vi "Joint Saturation.vi"(10 "Joint Bounds [Deg/mm]":dbl[][](array[numeric])=[[-10.0, 35.0, 0.0, 0.0], [-35.0, -35.0, 0.0, 0.0], [0.5, 10.0, 0.0, 0.0], [-40.0, 40.0, 0.0, 0.0]], 11 "Ref Array [Deg/mm]":dbl[](array[numeric])=[0.0, 0.0, 0.0, 0.0]) -> (3 "Sat Ref Array [Deg/mm]":dbl[](array[numeric]))   [LabVIEW 2016]
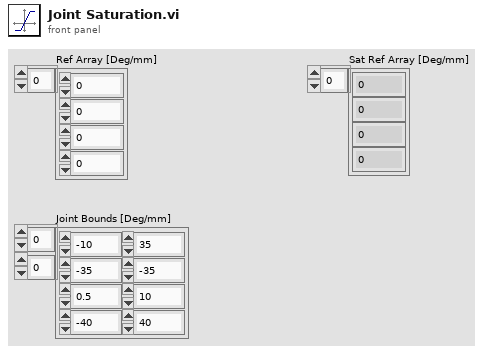
[diagram p1: front panel]
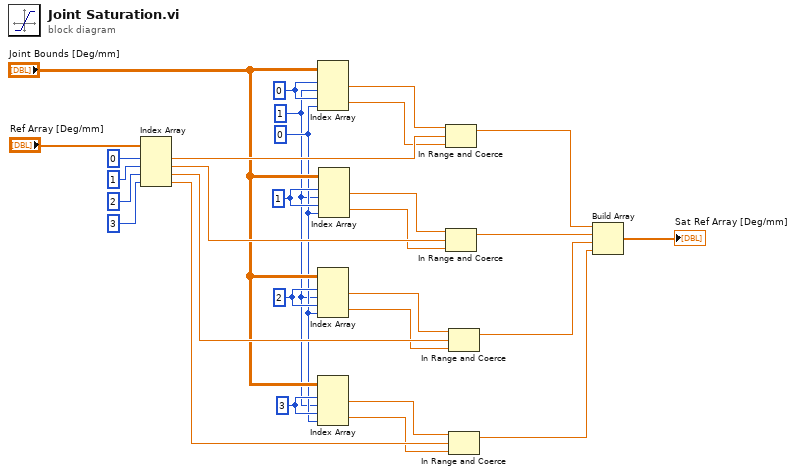
[diagram p0: block diagram]
diagram:
  w5 = 3 ("index (row)")
  w9 = 2
  w16 = 1 ("index (row)")
  w3 = 1 ("disabled index (col)")
  w4 = 0 ("index")
  w20 = 0 ("index")
  n1 = Index Array(array="Ref Array [Deg/mm]", index #1=0 ("index"), index #2=1 ("index"), index #3=2 ("index"), index #4=3 ("index")) -> (element #1=w24:dbl, element #2=w23:dbl, element #3=w22:dbl, element #4=w21:dbl)
  n2 = Index Array(array="Joint Bounds [Deg/mm]", index (row) #1=w20, index (col) #1=w3, index (row) #2=w20, index (col) #2=w4) -> (element #1=w19:dbl, element #2=w18:dbl)
  n3 = Index Array(array="Joint Bounds [Deg/mm]", index (row) #1=w9, index (col) #1=w3, index (row) #2=w9, index (col) #2=w4) -> (element #1=w8:dbl, element #2=w7:dbl)
  n4 = Index Array(array="Joint Bounds [Deg/mm]", index (row) #1=w5, index (col) #1=w3, index (row) #2=w5, index (col) #2=w4) -> (element #1=w2:dbl, element #2=w1:dbl)
  n5 = Index Array(array="Joint Bounds [Deg/mm]", index (row) #1=w16, index (col) #1=w3, index (row) #2=w16, index (col) #2=w4) -> (element #1=w15:dbl, element #2=w14:dbl)
  n6 = In Range and Coerce(upper limit=w19, x=w24, lower limit=w18) -> (coerced(x)=w17:dbl)  [unwired: 1 out]
  n7 = In Range and Coerce(upper limit=w15, x=w23, lower limit=w14) -> (coerced(x)=w12:dbl)  [unwired: 1 out]
  n8 = In Range and Coerce(upper limit=w8, x=w22, lower limit=w7) -> (coerced(x)=w11:dbl)  [unwired: 1 out]
  n9 = In Range and Coerce(upper limit=w2, x=w21, lower limit=w1) -> (coerced(x)=w10:dbl)  [unwired: 1 out]
  n10 = Build Array(w17, w12, w11, w10) -> (→"Sat Ref Array [Deg/mm]":dbl[])
